vi "Main.vi"() -> ()   [LabVIEW 2023]
uses:
  ChildSink/ChildSink.lvclass
  ChildSource/ChildSource.lvclass
  PropertyBinder/PropertyBinder.lvclass
  PropertyBinder/PropertyBinder.lvclass/PropertyBinder.ctl
  b163268c-942b-43dd-84ea-4c1a13c0b956.vi
  PropertyBinder/GetSourceGetter.vi
  PropertyBinder/GetGetterAccessorInfo.vi
  PropertyBinder/GetSetterAccessorInfo.vi
  PropertyBinder/GetSinkSetter.vi
panel:
  out "Data":dbl
  out "x = y?":bool
  out "UpdatedSink":refnum<class "ChildSink.lvclass">
  out "error out":errorcluster
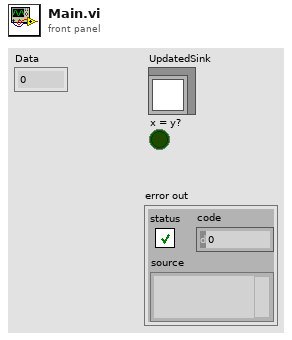
[diagram p1: front panel]
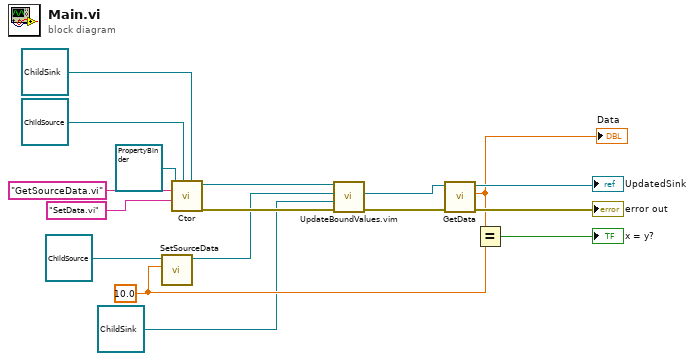
[diagram p0: block diagram]
diagram:
  w5 = 10.0 ("SourceData")
  n1 = call-dynamic "SetSourceData.vi"("SourceData"=w5, "ChildSource in"=refnum<class "ChildSource.lvclass"> refnum ("ChildSource.lvclass")) -> ("ChildSource out"=w9:refnum<class "ChildSource.lvclass">)  [unwired: 8 in, 1 out]
  n2 = call "Ctor.vi"("SinkType"=refnum<class "ChildSink.lvclass"> refnum ("ChildSink.lvclass"), "SourceType"=refnum<class "ChildSource.lvclass"> refnum ("ChildSource.lvclass"), "SinkSetter"="SetData.vi", "SourceGetter"="GetSourceData.vi", "PropertyBinder"=refnum<class "PropertyBinder.lvclass"> refnum) -> ("error out"=w12:errorcluster, "PropertyBinder"=w13:refnum<class "PropertyBinder.lvclass">)  [unwired: 5 in]
  n3 = call "UpdateBoundValues.vim"("error in (no error)"=w12, "Sink"=refnum<class "ChildSink.lvclass"> refnum ("ChildSink.lvclass"), "Source"=w9, "PropertyBinder in"=w13) -> ("error out"=w1:errorcluster, "UpdatedSink"=w2:refnum<class "ChildSink.lvclass">)  [unwired: 5 in, 1 out]
  n4 = call-dynamic "GetData.vi"("error in (no error)"=w1, "ChildSink in"=w2) -> ("error out"=→"error out":errorcluster, "Data"=w6:dbl, "ChildSink out"=→"UpdatedSink":refnum<class "ChildSink.lvclass">)  [unwired: 7 in]
  "Data" <- w6
  n5 = Equal?(x=w6, y=w5) -> (x = y?=→"x = y?":bool)
